vi "禁启用.vi"(10 "Enabled？":bool, 11 "数组":refnum<vi>[](array[refnum])) -> ()   [LabVIEW 2014]
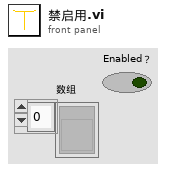
[diagram p1: front panel]
types:
  T1 = enum8{"Enabled", "Disabled", "Disabled and Grayed Out"}
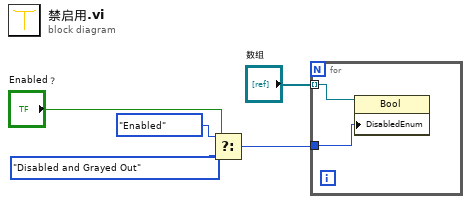
[diagram p0: block diagram]
diagram:
  n1 = Select(t=T1."Enabled" ("禁用"), s="Enabled？", f=T1."Disabled and Grayed Out") -> (s? t:f=w3:T1)
  n2 = for {
    tunnel: "数组" -> [w7] mode=indexing
    tunnel: w3 -> [w6]
    n3 = property class="Bool"(reference=w7, "DisabledEnum"=w6) -> ()  [unwired: 1 in, 2 out]
  }
